vi "update coordinates from center even.vi"(8 "error in (no error)":errorcluster caption="错误输入（无错误）", 9 "Radial size":i32, 10 "center_y":i32, 11 "center_x":i32) -> (0 "error out":errorcluster caption="错误输出", 2 "CoordinatesOut":i32[](array[numeric]))   [LabVIEW 2013]
panel:
  in  "Y上限":i32=493
  in  "X_上限":i32=659
  out "范围出错":bool
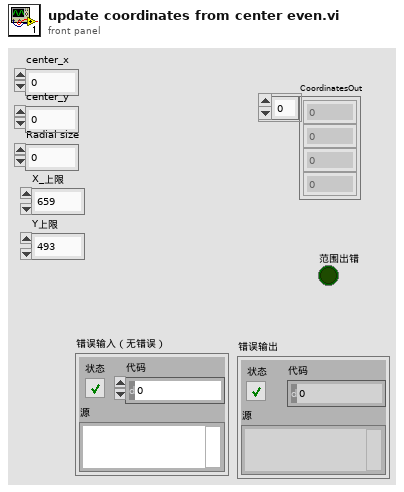
[diagram p1: front panel]
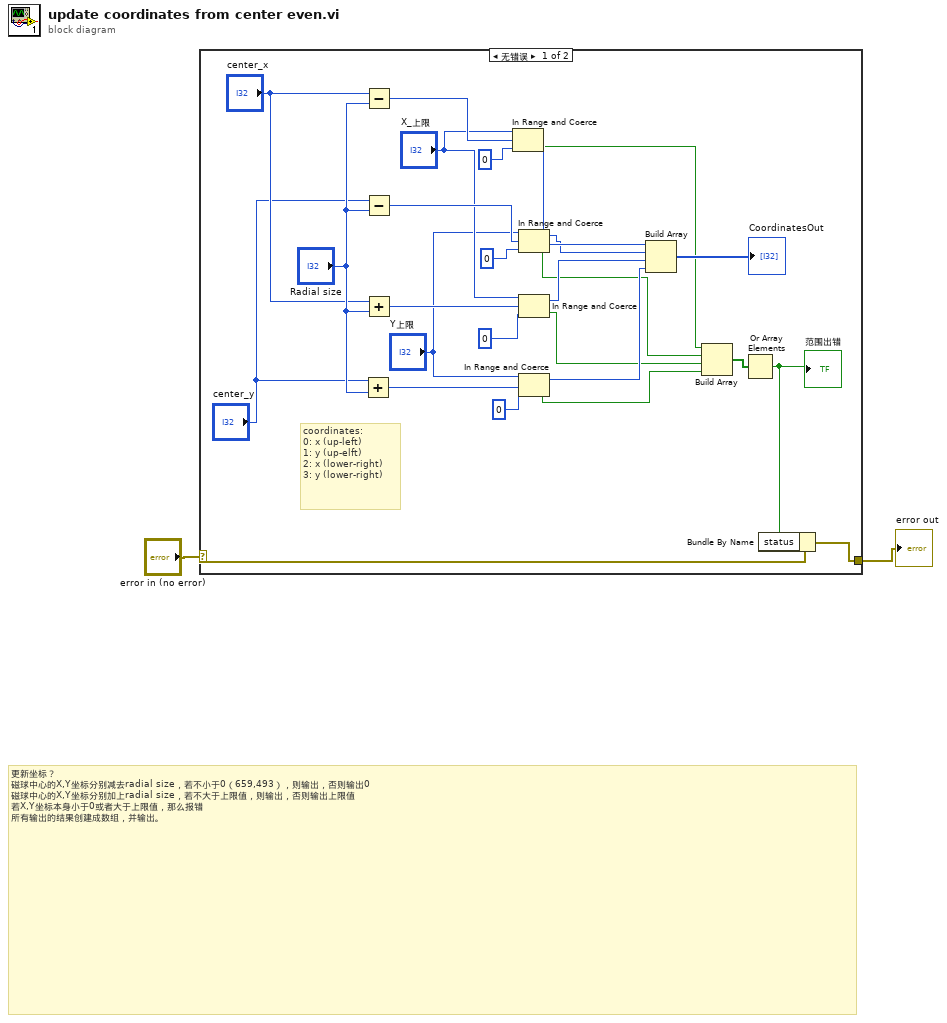
[diagram p0: block diagram]
diagram:
  # "更新坐标？\n磁球中心的X,Y坐标分别减去radial size，若不小于0（659,493），则输出，否则输出0\n磁球中心的X,Y坐标分别加上radial size，若不大于上限值，则输出，否则输出上限值\n若X,Y坐标本身小于0或者大于上限值，那么报错\n所有输出的结果创建成数组，并输出。"
  n1 = case shown="无错误" "error in (no error)" {
    selector: "error in (no error)" -> [w7 w29]
    tunnel: [w5 w29] -> w1
    frame No Error {
      # "coordinates:\n0: x (up-left)\n1: y (up-elft)\n2: x (lower-right)\n3: y (lower-right)"
      n2 = Add(x="center_y", y="Radial size") -> (x+y=w18:i32)
      n3 = Subtract(x="center_x", y="Radial size") -> (x-y=w24:i32)
      n4 = Subtract(x="center_y", y="Radial size") -> (x-y=w22:i32)
      n5 = Add(x="center_x", y="Radial size") -> (x+y=w17:i32)
      n6 = In Range and Coerce(upper limit="X_上限", x=w24, lower limit=0 ("下限")) -> (coerced(x)=w16:i32, In Range?=w12:bool)
      n7 = In Range and Coerce(upper limit="Y上限", x=w22, lower limit=0 ("下限")) -> (coerced(x)=w15:i32, In Range?=w11:bool)
      n8 = In Range and Coerce(upper limit="X_上限", x=w17, lower limit=0 ("下限")) -> (coerced(x)=w14:i32, In Range?=w10:bool)
      n9 = In Range and Coerce(upper limit="Y上限", x=w18, lower limit=0 ("下限")) -> (coerced(x)=w13:i32, In Range?=w9:bool)
      n10 = Build Array(w16, w15, w14, w13) -> (→"CoordinatesOut":i32[])
      n11 = Build Array(w12, w11, w10, w9) -> (w8:bool[])
      n12 = Or Array Elements(Boolean array=w8) -> (logical OR=w6:bool)
      "范围出错" <- w6
      n13 = Bundle By Name(cluster=w7, "status"=w6) -> (w5:errorcluster)
    }
    frame Error {
    }
  }
  "error out" <- w1
